vi "TestDataConverstionToMatlab.vi"() -> ()   [LabVIEW 2017]
uses:
  Types/MatlabDataBundle.ctl
  Types/MatlabDataType.ctl
  Types/ScanInfo.ctl
panel:
  in  "Waveform":waveform(dbl)
  out "data":dbl[][](array[numeric])
  in  "Position":cluster{"X":dbl, "Y":dbl} {"Y" step=0.01; "X" step=0.01}
  in  "ScanConfig":T1={"X"=0.0, "Y"=0.0, "Width"=1.0, "Height"=1.0, "Time"=1000.0, "AsDwellTime"=FALSE, "N"=1000.0, "FromCenter"=TRUE}
  in  "Somename":string="Lama"
  in  "Read Back from matlab":bool=TRUE
  out "Curent exec pos":string="read data"
  out "erros?":bool
  in  "milliseconds to wait":u32
  in  "Single Run":bool
  in  "Do convert back":bool=TRUE
  in  "Convert \nThrough \nMatlab":bool=TRUE
  out "Matlab param info":T2[](array[typedef])=[{"MatlabType"=enum."Real", "Value"=variant(dbl 0.0), "Name"="SimpleCluster@X", "Typename"="real"}, {"MatlabType"=enum."Real", "Value"=variant(dbl 0.0), "Name"="SimpleCluster@Y", "Typename"="real"}, {"MatlabType"=enum."String", "Value"=variant(string ""), "Name"="SimpleCluster@Somename", "Typename"="string"}]
  out "original":variant=variant(cluster{"X":dbl, "Y":dbl, "Somename":string} {"X"=2.0, "Y"=3.0, "Somename"="Lama"})
  out "After converstion back":variant=variant(cluster{"X":dbl, "Y":dbl, "Somename":string} {"X"=0.0, "Y"=0.0, "Somename"=""})
  in  "Multidim3d":dbl[][][](array[numeric])=[[[1.0, 2.0], [1.0, 2.0]], [[1.0, 2.0], [1.0, 2.0]]]
  in  "Multidim2d":dbl[][](array[numeric])=[[1.0, 2.0], [1.0, 2.0]]
  in  "TestDataBunch":cluster{"Data":dbl[]}[](array[cluster])=[{"Data"=[1.0, 2.0, 3.0]}, {"Data"=[4.0, 5.0, 6.0]}, {"Data"=[7.0, 8.0, 9.0]}]
  out "ExpID":string="Exp77c27ca2690b43b31b68791e85e1b449C"
  in  "Array of clusters Convert":cluster{"A":dbl, "B":dbl}[](array[cluster])=[{"A"=1.0, "B"=2.0}, {"A"=3.0, "B"=4.0}, {"A"=5.0, "B"=6.0}]
  in  "Simple":dbl=55.0
  out "Params Size":i32=3
  in  "SomeContainer":cluster{"TheArray":cluster{"A":dbl, "B":dbl}[]}={"TheArray"=[{"A"=1.0, "B"=2.0}, {"A"=3.0, "B"=4.0}, {"A"=5.0, "B"=6.0}]}
  in  "Onedim":dbl[](array[numeric])=[1.0, 2.0, 3.0, 4.0, 5.0]
  in  "SimpleCluster":cluster{"X":dbl, "Y":dbl, "Somename":string}={"X"=2.0, "Y"=3.0, "Somename"="Lama"}
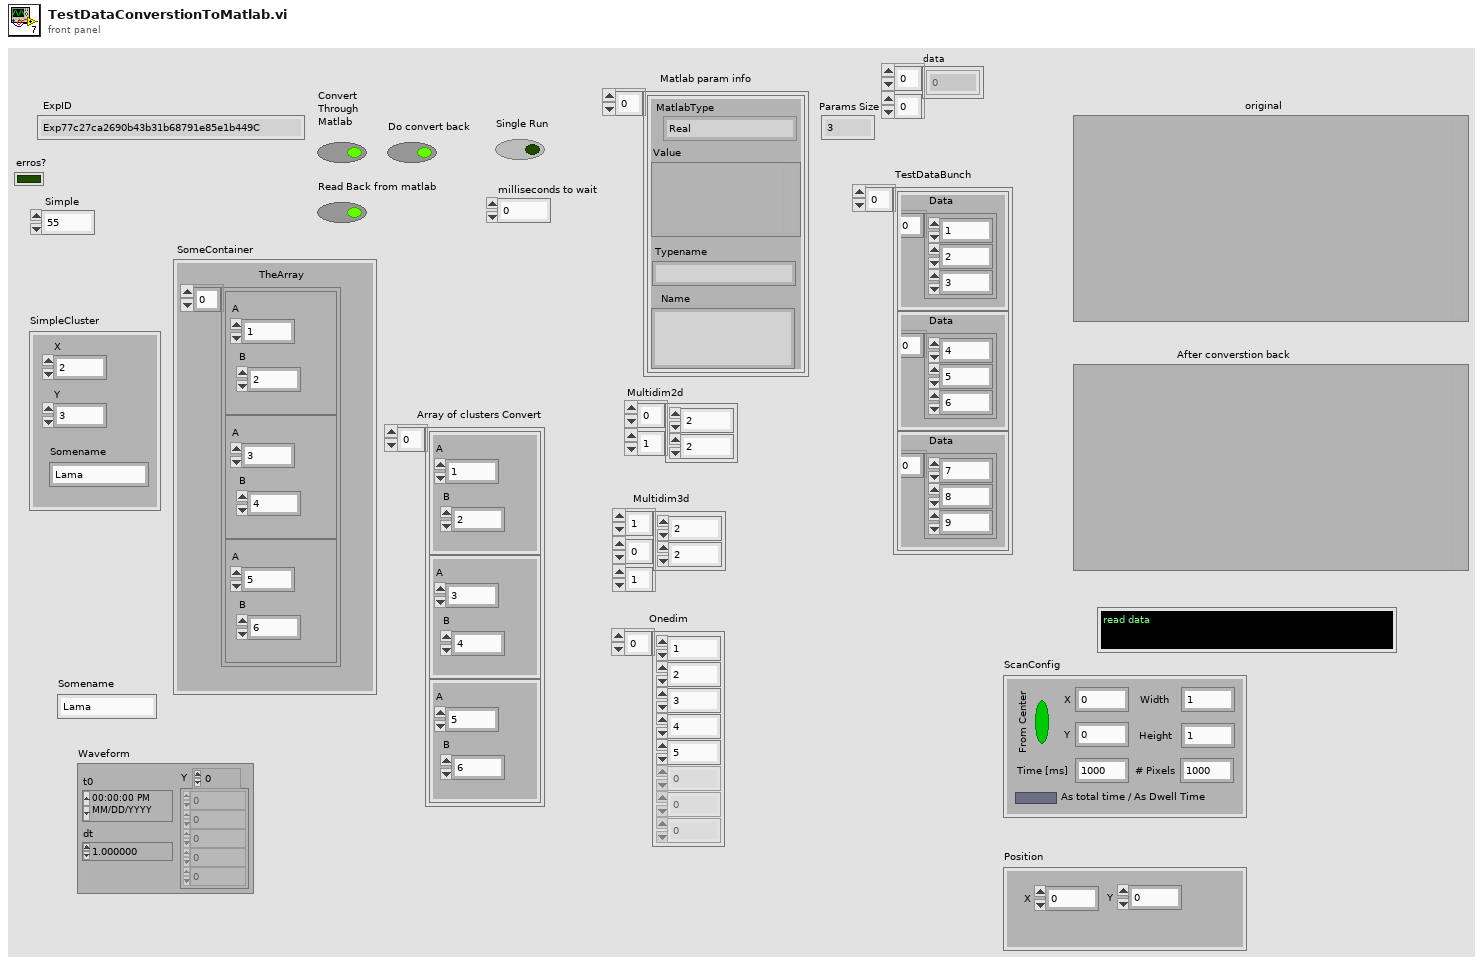
[diagram p1: front panel]
types:
  T1 = typedef "ScanInfo.ctl" = cluster{"X":dbl, "Y":dbl, "Width":dbl, "Height":dbl, "Time":dbl, "AsDwellTime":bool, "N":dbl, "FromCenter":bool}
  T2 = typedef "MatlabDataBundle.ctl" = cluster{"MatlabType":T3, "Value":variant, "Name":string, "Typename":string}
  T3 = typedef "MatlabDataType.ctl" = enum16{"NotAMatlabType", "Real", "Complex", "String", "Boolean"}
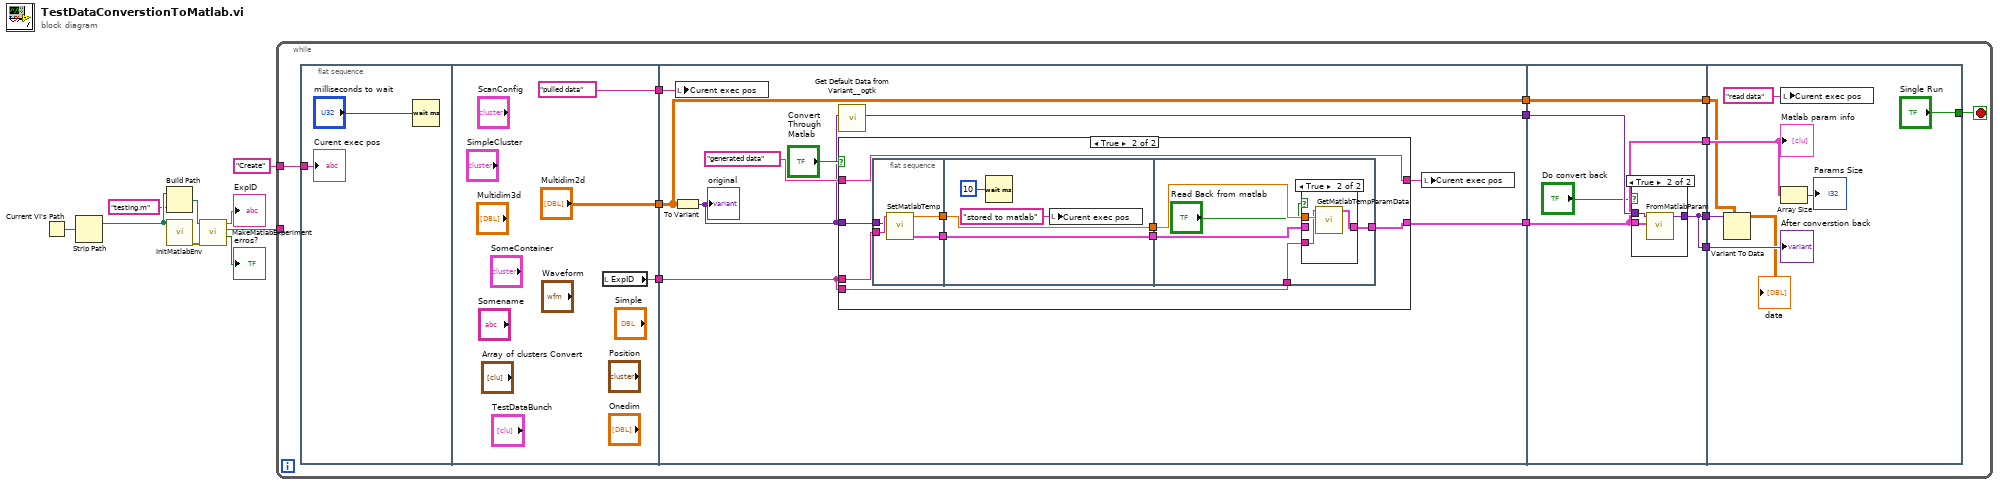
[diagram p0: block diagram]
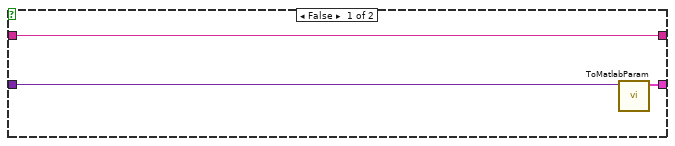
[diagram p2: hidden frame]
diagram:
  n1 = Current VI's Path() -> (path=w6:path)
  n2 = Strip Path(path=w6) -> (stripped path=w8:path)  [unwired: 1 out]
  n3 = Build Path(base path=w8, name or relative path="testing.m") -> (appended path=w9:path)
  n4 = call "InitMatlabEnv.vi"("Working directory"=w8) -> ("error out"=w7:errorcluster)  [unwired: 10 in]
  n5 = call "MakeMatlabExperiment.vi"("error in"=w7, "experimentFilepath"=w9) -> ("erros?"=→"erros?":bool, "errors"=w2:string, "ExpID"=→"ExpID":string)  [unwired: 6 in, 1 out]
  n6 = while {
    tunnel: w2 -> [_]
    tunnel: "Create" ("Curent exec pos") -> [w11]
    stop <- w20 stop-if-true
    n7 = flat-sequence {
      tunnel: w11 -> [w22]
      tunnel: [w26] -> w21
      tunnel: ["pulled data" ("Curent exec pos")] -> w13
      tunnel: ["Multidim2d"] -> w10
      tunnel: [w30] -> w18
      tunnel: [w28] -> w15
      tunnel: w21 -> [w31]
      tunnel: w13 -> [w32]
      tunnel: [w29] -> w12
      tunnel: w10 -> [w28]
      tunnel: [w66] -> w19
      tunnel: w18 -> [w67]
      tunnel: [w67] -> w17
      tunnel: [w66] -> w16
      tunnel: w15 -> [w69]
      tunnel: [w69] -> w14
      tunnel: w12 -> [w68]
      tunnel: w19 -> [w79]
      tunnel: w17 -> [w80]
      tunnel: w16 -> [w78]
      tunnel: w14 -> [w77]
      tunnel: ["Single Run"] -> w20
      frame #0 {
        n8 = Wait (ms)(milliseconds to wait="milliseconds to wait") -> ()  [unwired: 1 out]
        "Curent exec pos" <- w22
      }
      frame #1 {
        n9 = local read "ExpID"() -> (w26:string)
      }
      frame #2 {
        n10 = To Variant(anything=w28) -> (Variant=w27:variant)
        "original" <- w27
        n11 = local write "Curent exec pos"(w32) -> ()
        n12 = call <userlib>:"Get Default Data from Variant__ogtk.vi"("Variant"=w27) -> ("Default VData"=w29:variant)  [unwired: 9 in, 1 out]
        n13 = case shown="True" "Convert \nThrough \nMatlab" {
          tunnel: w27 -> [w38 w47]
          tunnel: w31 -> [_ w46]
          tunnel: "generated data" ("Curent exec pos") -> [w37 w45]
          tunnel: [w37 w45] -> w33
          tunnel: w31 -> [_ w44]
          tunnel: [w36 w43] -> w30
          frame False {
            n14 = call "ToMatlabParam.vi"("Value"=w38) -> ("Matlab Param Data"=w36:T2[])  [unwired: 10 in]
          }
          frame True {
            n15 = flat-sequence {
              tunnel: w47 -> [w48]
              tunnel: w46 -> [w51]
              tunnel: [w50] -> w42
              tunnel: [w49] -> w39
              tunnel: w42 -> [w55]
              tunnel: [w55] -> w41
              tunnel: [w53] -> w40
              tunnel: w39 -> [w53]
              tunnel: w41 -> [w60]
              tunnel: w44 -> [w59]
              tunnel: [w58] -> w43
              tunnel: w40 -> [w57]
              frame #0 {
                n16 = call "SetMatlabTemp.vi"("Variant"=w48, "ExpID"=w51) -> ("Matlab Param Data"=w49:T2[], "index out"=w50:dbl)  [unwired: 8 in]
              }
              frame #1 {
                n17 = Wait (ms)(milliseconds to wait=u32 10) -> ()  [unwired: 1 out]
                n18 = local write "Curent exec pos"("stored to matlab" ("Curent exec pos")) -> ()
              }
              frame #2 {
                n19 = case shown="True" "Read Back from matlab" {
                  tunnel: w60 -> [_ w64]
                  tunnel: w59 -> [_ w63]
                  tunnel: [w61 w62] -> w58
                  tunnel: w57 -> [w61 _]
                  frame False {
                  }
                  frame True {
                    n20 = call "GetMatlabTempParamData.vi"("index"=w64, "ExpID"=w63) -> ("Matlab param data"=w62:T2[])  [unwired: 9 in]
                  }
                }
              }
            }
          }
        }
        n21 = local write "Curent exec pos"(w33) -> ()
      }
      frame #3 {
        n22 = case shown="True" "Do convert back" {
          tunnel: w68 -> [w70 w73]
          tunnel: [w70 w72] -> w66
          tunnel: w67 -> [_ w71]
          frame False {
          }
          frame True {
            n23 = call "FromMatlabParam.vi"("Matlab Param Data"=w71, "Type (or value to update)"=w73) -> ("Value"=w72:variant)  [unwired: 9 in]
          }
        }
      }
      frame #4 {
        n24 = Variant To Data(type=w77, Variant=w78) -> (data=→"data":dbl[][])  [unwired: 1 in, 1 out]
        n25 = local write "Curent exec pos"("read data" ("Curent exec pos")) -> ()
        n26 = Array Size(array=w80) -> (size(s)=→"Params Size":i32)
        "Matlab param info" <- w80
        "After converstion back" <- w79
      }
    }
  }
